vi "LVtoJSON-DBInsert.vi"(4 "Type Of Insertion":i32, 5 "SQL Query Statement":string, 6 "Payload":string="Inventory", 7 "Update All":bool, 8 "error in":errorcluster, 9 "Columns":string[](array[string]), 10 "SQL Statement":string, 11 "Table":string="Inventory") -> (0 "error out":errorcluster, 3 "Output JSON Object":string)   [LabVIEW 2014]
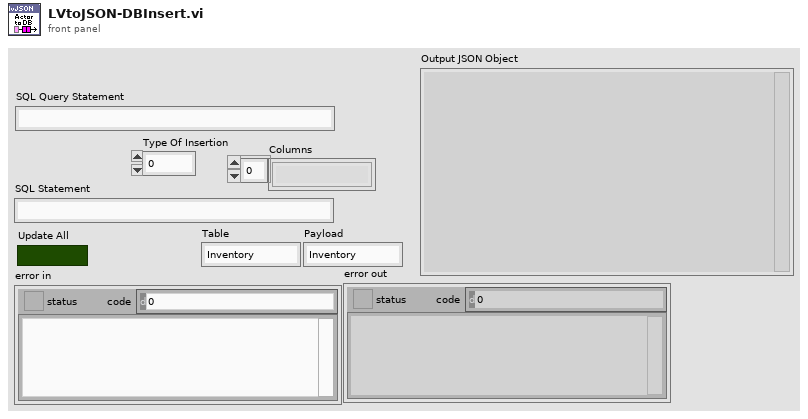
[diagram p1: front panel]
types:
  T1 = cluster{"Table":string, "SQL Statement":string, "Update All":bool, "Payload":string, "Type Of Insertion":i32, "SQL Query Statement":string, "Columns":string}
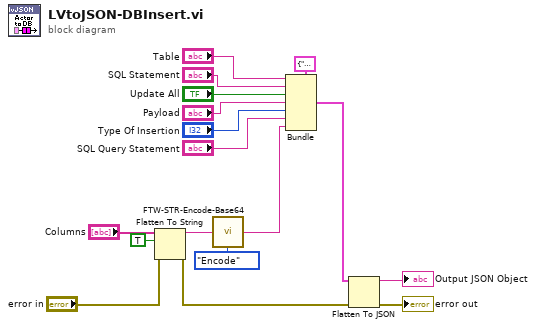
[diagram p0: block diagram]
diagram:
  n1 = Flatten To String(anything="Columns", prepend array or string size? (T)=TRUE, error in (no error)="error in") -> (data string=w6:string, error out=w3:errorcluster)  [unwired: 1 in, 1 out]
  n2 = call "FTW-STR-Encode-Base64.vi"("Input"=w6, "Direction"=enum16{"Encode", "Decode"}."Encode") -> ("Output"=w2:string)
  n3 = Bundle(cluster=T1 {"Table"="", "SQL Statement"="", "Update All"=FALSE, "Payload"="", "Type Of Insertion"=0, "SQL Query Statement"="", "Columns"=""}, "Table"="Table", "SQL Statement"="SQL Statement", "Update All"="Update All", "Payload"="Payload", "Type Of Insertion"="Type Of Insertion", "SQL Query Statement"="SQL Query Statement", "Columns"=w2) -> (w9:T1)
  n4 = Flatten To JSON(anything=w9, error in (no error)=w3) -> (JSON string=→"Output JSON Object":string, 11:→"error out":errorcluster)  [unwired: 1 in]
